vi "作业6 .vi"() -> ()   [LabVIEW 2017]
panel:
  in  "停止 2":bool
  out "显示面板":T1 {"油量" scale=0.0..10.0; "转速（转/秒）" scale=0.0..10000.0; "时速（公里/小时）" scale=0.0..280.0}
  in  "控制面板":T2 {"档位" scale=0.0..10.0; "油门" scale=0.0..100.0}
  out "鞍点":string
  out "随机数数组":dbl[][](array[numeric])
  out "字符串":string
  in  "开启报警":bool
  in  "停止":bool
  out "报警灯":bool
  out "温度计":dbl(slide) scale=0.0..100.0
  in  "报警上线":dbl(slide) scale=0.0..100.0
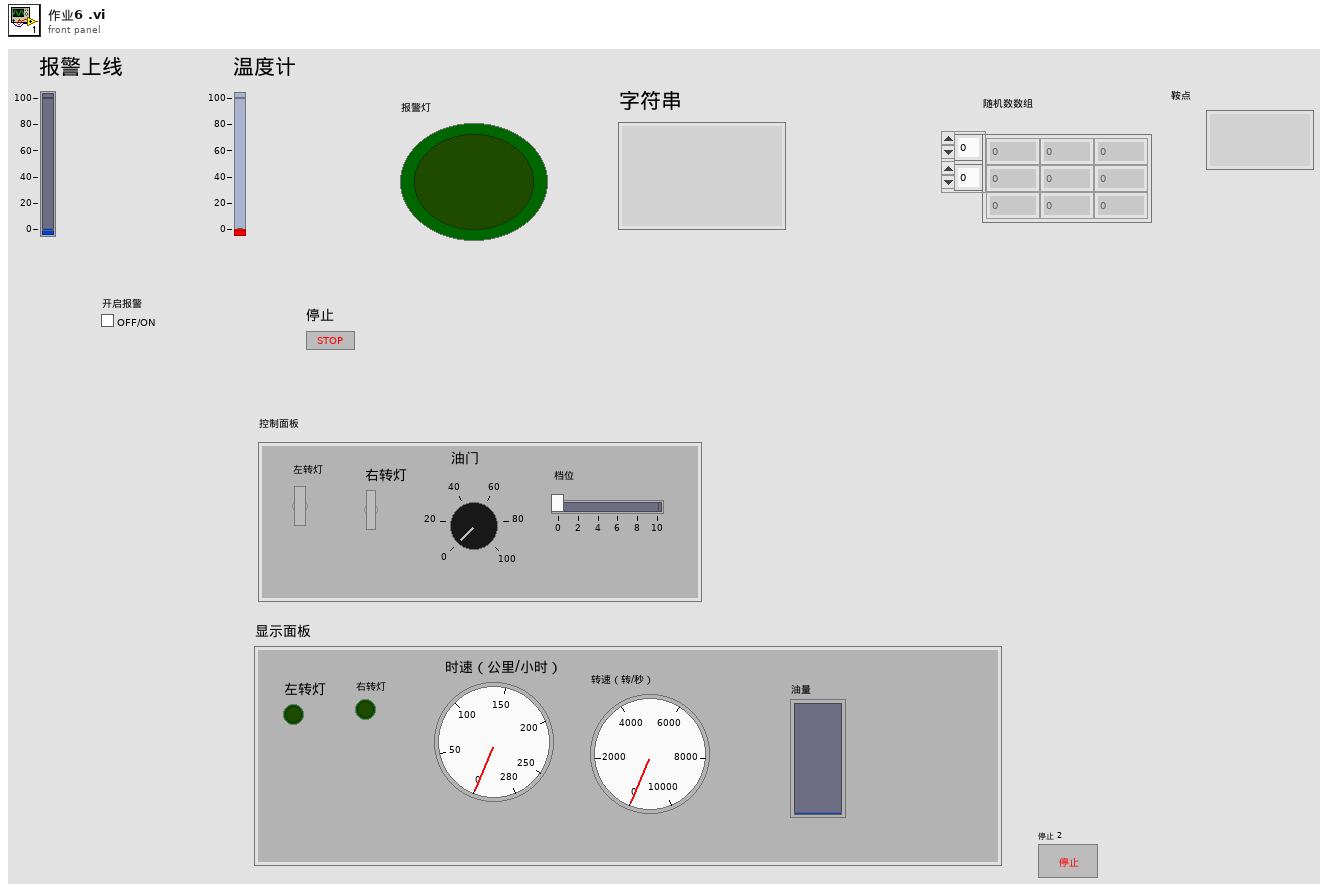
[diagram p1: front panel]
types:
  T1 = cluster{"左转灯":bool, "右转灯":bool, "时速（公里/小时）":dbl, "转速（转/秒） ":dbl, "油量":dbl}
  T2 = cluster{"左转灯":bool, "右转灯":bool, "油门":dbl, "档位":dbl}
  T3 = cluster{"左转灯":bool, "右转灯":bool, dbl, dbl, "b":dbl}
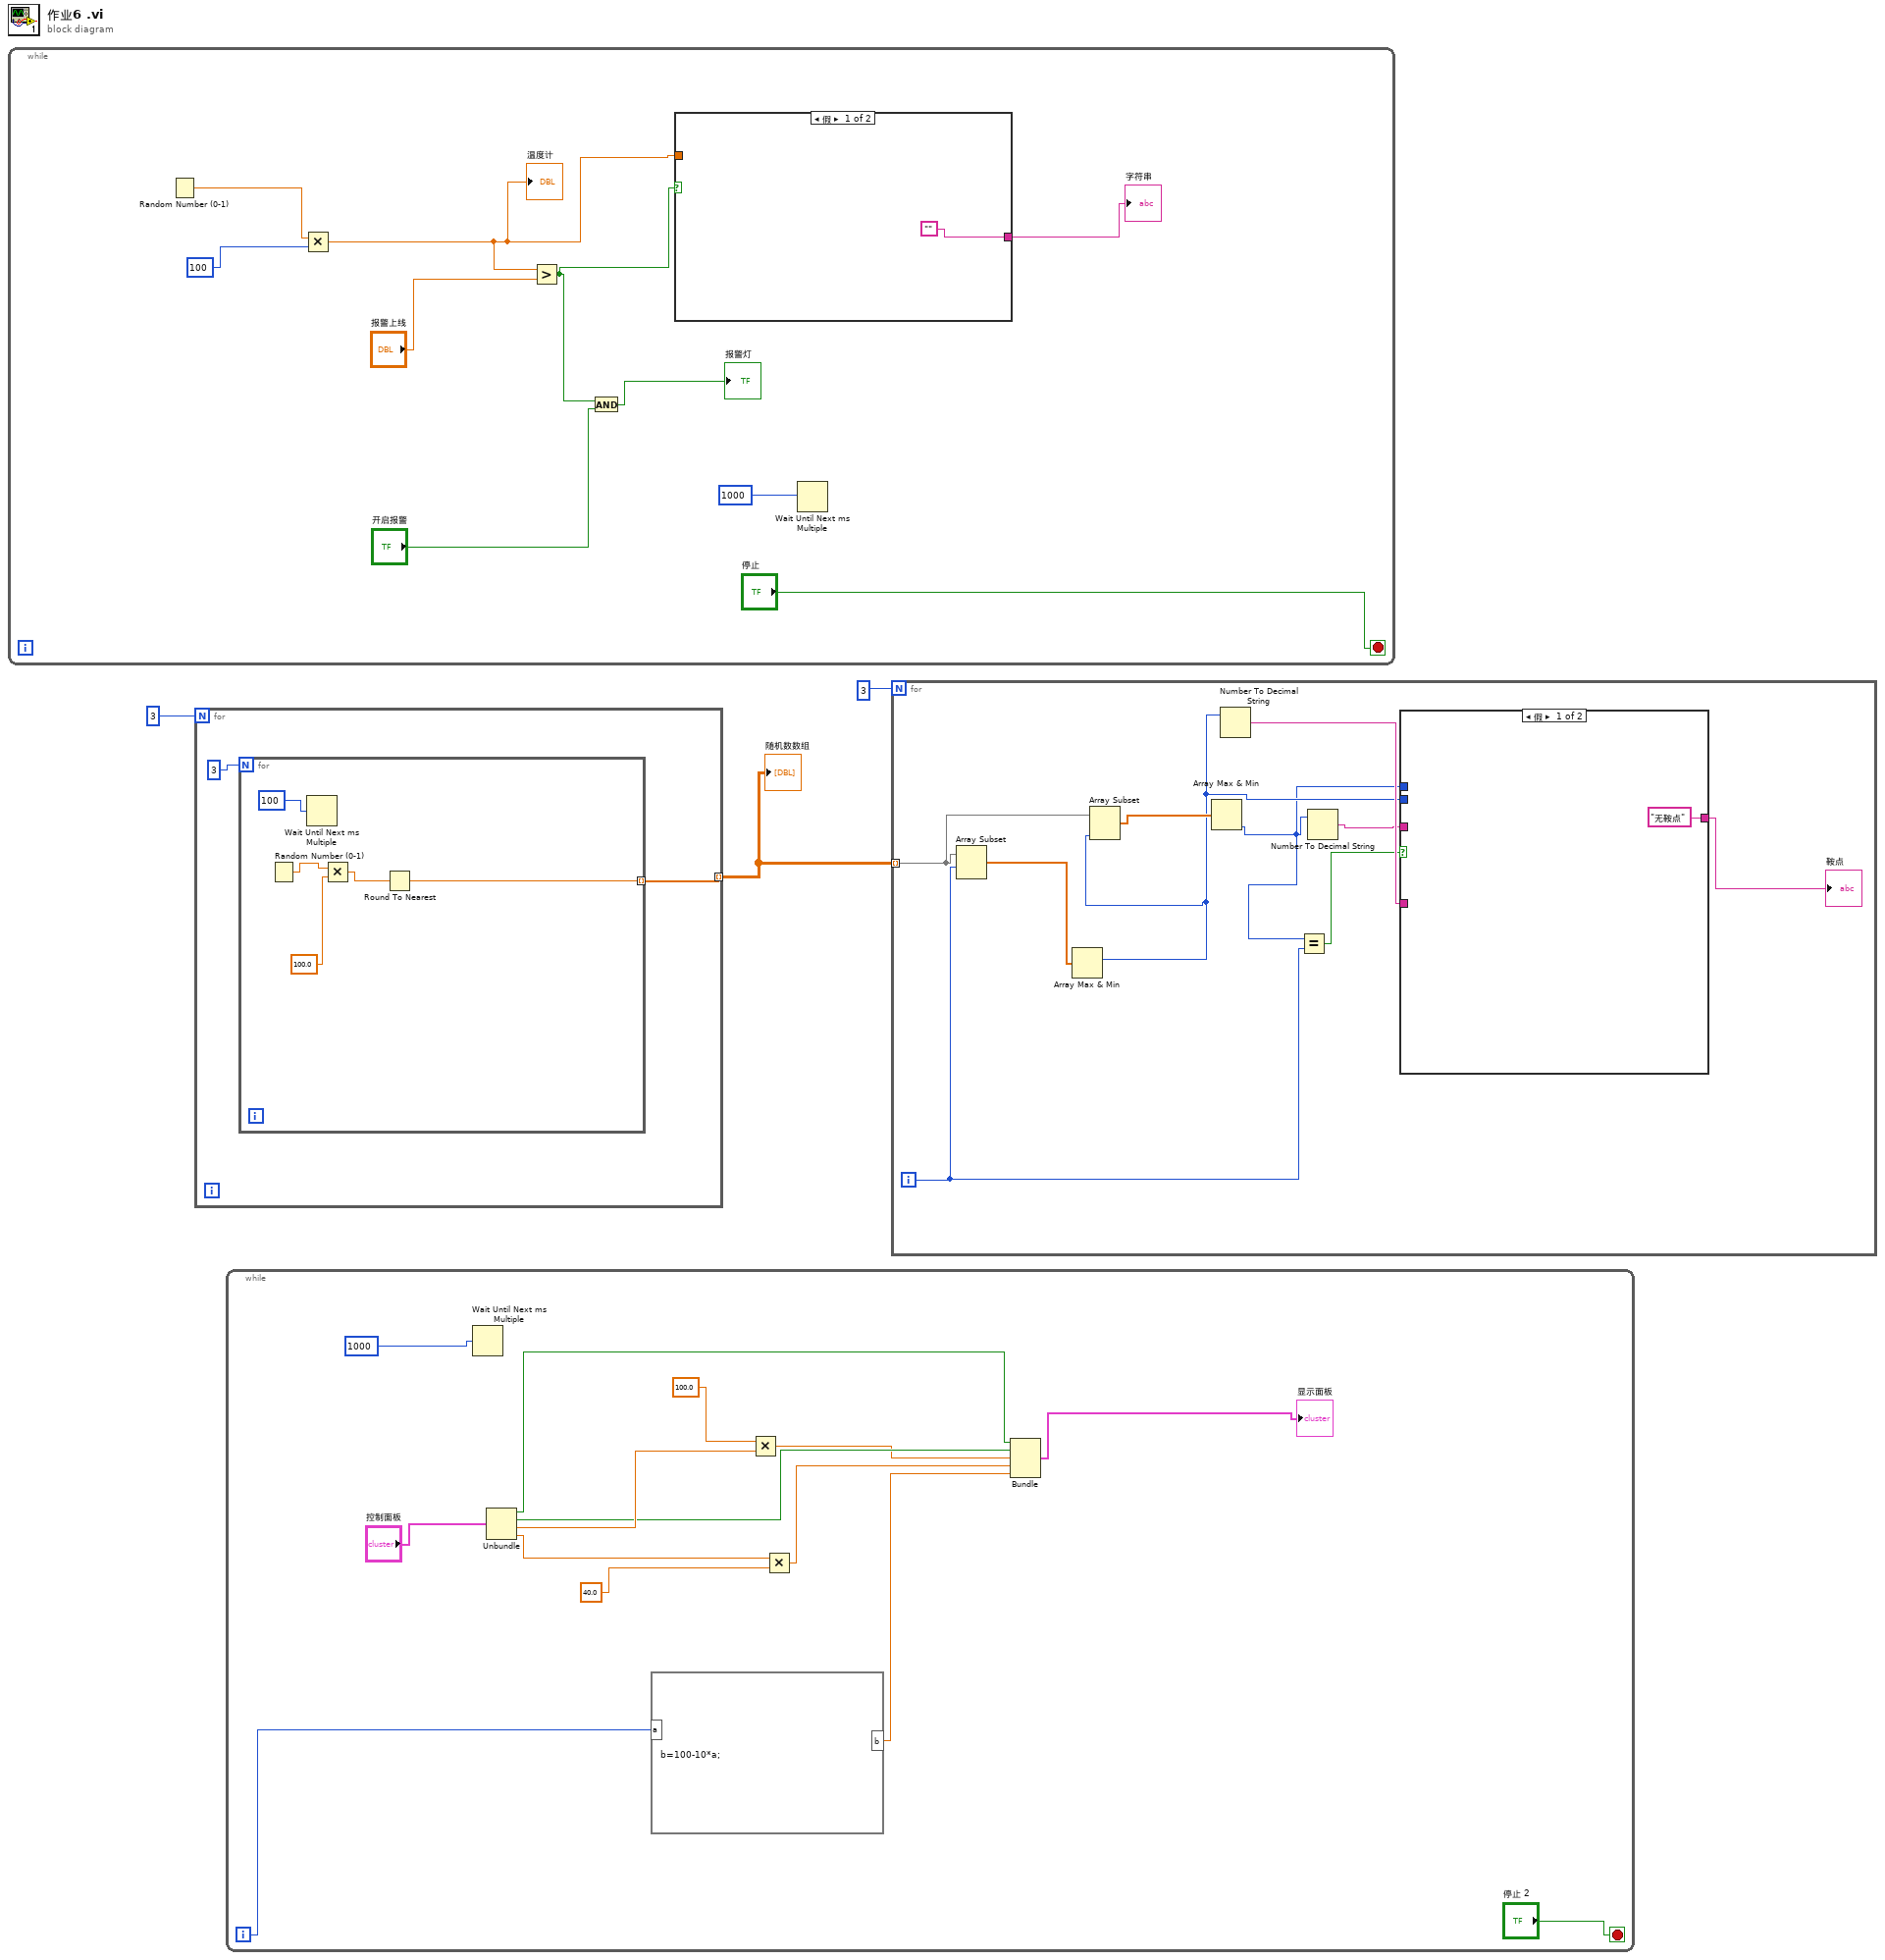
[diagram p0: block diagram]
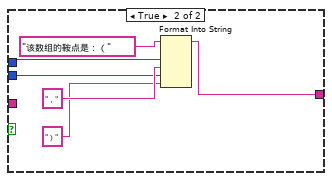
[diagram p2: hidden frame]
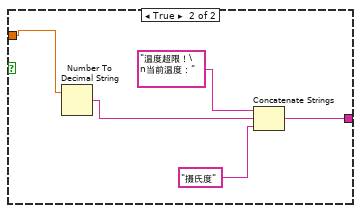
[diagram p3: hidden frame]
diagram:
  n1 = while {
    stop <- "停止" stop-if-true
    n2 = Random Number (0-1)() -> (number: 0 to 1=w9:dbl)
    n3 = Multiply(x=w9, y=100) -> (x*y=w11:dbl)
    "温度计" <- w11
    n4 = Greater?(x=w11, y="报警上线") -> (0:w4:bool)
    n5 = And(x=w4, y="开启报警") -> (x .and. y?=→"报警灯":bool)
    n6 = case shown="假" w4 {
      tunnel: w11 -> [_ w16]
      tunnel: ["" w15] -> w5
      frame False {
      }
      frame True {
        n7 = Number To Decimal String(number=w16) -> (decimal integer string=w18:string)  [unwired: 1 in]
        n8 = Concatenate Strings("温度超限！\n当前温度：", w18, "摄氏度") -> (w15:string)
      }
    }
    "字符串" <- w5
    n9 = Wait Until Next ms Multiple(millisecond multiple=1000) -> ()  [unwired: 1 out]
  }
  n10 = for {
    N: 3 -> [_]
    tunnel: [w20] -> w3 mode=indexing
    n11 = for {
      N: 3 -> [_]
      tunnel: [w22] -> w20 mode=indexing
      n12 = Random Number (0-1)() -> (number: 0 to 1=w25:dbl)
      n13 = Wait Until Next ms Multiple(millisecond multiple=100) -> ()  [unwired: 1 out]
      n14 = Multiply(x=w25, y=100.0) -> (x*y=w23:dbl)
      n15 = Round To Nearest(number=w23) -> (nearest integer value=w22:dbl)
    }
  }
  "随机数数组" <- w3
  n16 = while {
    i -> [w34]
    stop <- "停止 2" stop-if-true
    n17 = Wait Until Next ms Multiple(millisecond multiple=1000) -> ()  [unwired: 1 out]
    n18 = Unbundle("控制面板") -> ("左转灯"=w31:bool, "右转灯"=w28:bool, "油门"=w38:dbl, "档位"=w37:dbl)
    n19 = formula code="b=100-10*a;"("a"=w34) -> ("b"=w30:dbl)
    n20 = Multiply(x=100.0, y=w38) -> (x*y=w27:dbl)
    n21 = Multiply(x=w37, y=40.0) -> (x*y=w29:dbl)
    n22 = Bundle("左转灯"=w31, "右转灯"=w28, w27, w29, "b"=w30) -> (→"显示面板":T3)  [unwired: 1 in]
  }
  n23 = for {
    N: 3 -> [_]
    tunnel: w3 -> [w49] mode=indexing
    i -> [w47]
    n24 = Array Subset(array=w49, index=w47) -> (w50:dbl[])  [unwired: 1 in]
    n25 = Array Max & Min(array=w50) -> (max index (indices)=w44:i32)  [unwired: 3 out]
    n26 = Array Subset(array=w49, length=w44) -> (w48:dbl[])  [unwired: 1 in]
    n27 = Array Max & Min(array=w48) -> (min index (indices)=w42:i32)  [unwired: 3 out]
    n28 = Number To Decimal String(number=w44) -> (decimal integer string=w46:string)  [unwired: 1 in]
    n29 = Equal?(x=w42, y=w47) -> (x = y?=w45:bool)
    n30 = Number To Decimal String(number=w42) -> (decimal integer string=w43:string)  [unwired: 1 in]
    n31 = case shown="假" w45 {
      tunnel: w46 -> [_ _]
      tunnel: ["无鞍点" w54] -> w41
      tunnel: w44 -> [_ w53]
      tunnel: w43 -> [_ _]
      tunnel: w42 -> [_ w52]
      frame False {
      }
      frame True {
        n32 = Format Into String(initial string="该数组的鞍点是：（", w52, "，", w53, "）") -> (resulting string=w54:string)  [unwired: 2 in, 1 out]
      }
    }
    "鞍点" <- w41
  }
